vi "Cursor Redraw Write.vi"(4 "error in (no error)":errorcluster, 5 "Value":bool, 6 "Container State":T4, 7 "Display State In":T1={"Numeric"=0.0, "Timeline Ref"=refnum, "Waveform Ref"=refnum, "Fill Plots"=FALSE, "Cursor Redraw"=TRUE}) -> (0 "error out":errorcluster, 3 "Display State Out":T1={"Numeric"=0.0, "Timeline Ref"=refnum, "Waveform Ref"=refnum, "Fill Plots"=FALSE, "Cursor Redraw"=TRUE})   [LabVIEW 2020, in "XGrapher.xctl"]
uses:
  XGrapher.xctl
  <vilib>/_xctls/Container State.ctl
  State 1.ctl
  Typedefs/Xctrl-Timeline graph ref.ctl
  Typedefs/Xctrl-Waveform graph ref.ctl
  <vilib>/_xctls/XControlSupport.lvlib
panel:
  # "Replace the Value Control below with a Control of desired type.\nDo not remove this Control or the others from the connector pane.\nDo not change the connector pane pattern.\nThe Value control should always be the third terminal from top on the input side in the connector pane."
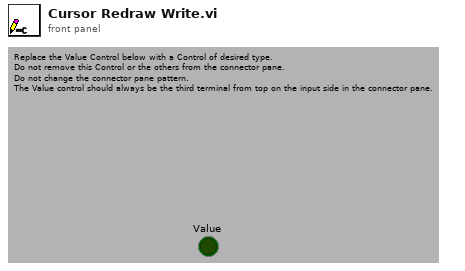
[diagram p1: front panel]
types:
  T1 = typedef "XGrapher.xctl/State 1.ctl" = cluster{"Numeric":dbl, "Timeline Ref":T2, "Waveform Ref":T3, "Fill Plots":bool, "Cursor Redraw":bool}
  T2 = typedef "XGrapher.xctl/Xctrl-Timeline graph ref.ctl" = refnum<vi>
  T3 = typedef "XGrapher.xctl/Xctrl-Waveform graph ref.ctl" = refnum<vi>
  T4 = typedef "XControlSupport.lvlib/Container State.ctl" = cluster{"Indicator?":bool, "Run Mode?":bool, " Refnum":refnum<vi>}
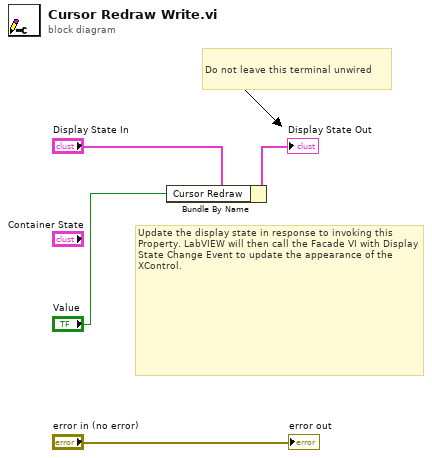
[diagram p0: block diagram]
diagram:
  # "Do not leave this terminal unwired"
  # "Update the display state in response to invoking this Property. LabVIEW will then call the Facade VI with Display State Change Event to update the appearance of the XControl."
  n1 = Bundle By Name(cluster="Display State In", "Cursor Redraw"="Value") -> (→"Display State Out":T1)
  "error out" <- "error in (no error)"
